vi "角度计算.vi"(10 "远心坐标":cluster{"X":sgl, "Y":sgl}, 11 "圆弧上三个点坐标":cluster{"X":dbl, "Y":dbl}[](array[cluster])) -> (3 "Angle":dbl[](array[numeric]))   [LabVIEW 2014]
uses:
  <vilib>/vision/NI_Vision_Development_Module.lvlib
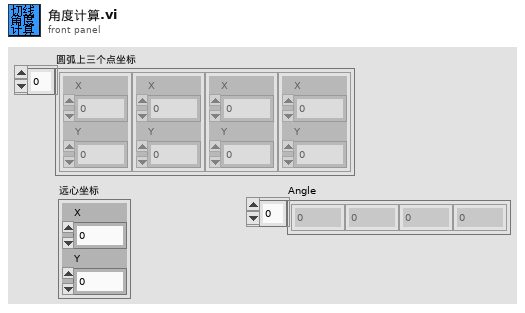
[diagram p1: front panel]
types:
  T1 = cluster{cluster{"X":dbl, "Y":dbl}, "远心坐标":cluster{"X":sgl, "Y":sgl}}
  T2 = cluster{"远心坐标":cluster{"X":sgl, "Y":sgl}, cluster{sgl, "Y":sgl}}
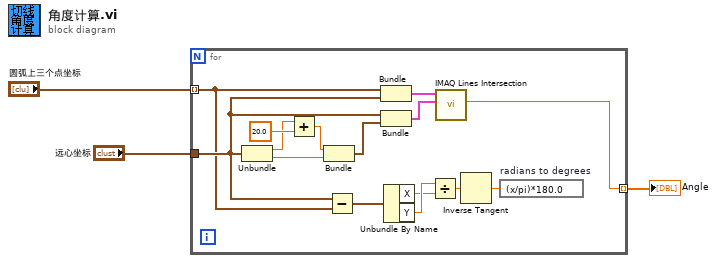
[diagram p0: block diagram]
diagram:
  n1 = for {
    tunnel: "远心坐标" -> [w11]
    tunnel: [w4] -> w1 mode=indexing
    tunnel: "圆弧上三个点坐标" -> [w10] mode=indexing
    n2 = Unbundle(w11) -> ("X"=w12:sgl, "Y"=w15:sgl)
    n3 = Add(x=w12, y=sgl 20.0) -> (x+y=w14:sgl)
    n4 = Bundle(w14, "Y"=w15) -> (w17:cluster{sgl, "Y":sgl})  [unwired: 1 in]
    n5 = Subtract(x=w11, y=w10) -> (x-y=w9:cluster{"X":dbl, "Y":dbl})
    n6 = Bundle(w10, "远心坐标"=w11) -> (w16:T1)  [unwired: 1 in]
    n7 = Bundle("远心坐标"=w11, w17) -> (w18:T2)  [unwired: 1 in]
    n8 = Unbundle By Name(w9) -> ("X"=w7:dbl, "Y"=w8:dbl)
    n9 = Divide(x=w8, y=w7) -> (x/y=w6:dbl)
    n10 = call "IMAQ Lines Intersection"("Line 2"=w18, "Line 1"=w16) -> ("Angle"=w4:dbl)  [unwired: 7 in, 2 out]
    n11 = Inverse Tangent(1:w6) -> (0:w5:dbl)
    n12 = expression code="(x/pi)*180.0" "radians to degrees"(w5) -> ()  [unwired: 1 out]
  }
  "Angle" <- w1
